vi "svx_DAQ_ConvertState_2000toCurrent.vi"(10 "State_2000":T8 {"Channel Info Array"."Channel Type" items=["Voltage (V)"=0, "Charge (C)"=9, "-"=99, "SPL (Pa)"=3, "Force (lbf)"=6, "Force (N)"=1, "Acceleration (g) - IEPE"=2, "Acceleration (g) - Charge"=12, "Acceleration (g) - 4 wire DC Voltage"=22, "Velocity (in/s)"=7, "Velocity (mm/s)"=8, "Prox Probe (mil)"=4, "Prox Probe (mm)"=5]}, 11 "Default Control State in":T9 caption="State" {"Timing Control 2" format="%#_6f"; "Channel Info Array"."Max" min=0.0 format="± %^#_4g"; "Channel Info Array"."Channel Type" items=["Voltage (V)"=0, "Charge (C)"=9, "-"=99, "SPL (Pa)"=3, "Force (lbf)"=6, "Force (N)"=1, "Acceleration (g) - IEPE"=2, "Acceleration (g) - Charge"=12, "Acceleration (g) - 4 wire DC Voltage"=22, "Velocity (in/s)"=7, "Velocity (mm/s)"=8, "Prox Probe (mil)"=4, "Prox Probe (mm)"=5]}) -> (3 "Default Control State out":T9 caption="State" {"Timing Control 2" format="%#_6f"; "Channel Info Array"."Max" min=0.0 format="± %^#_4g"; "Channel Info Array"."Channel Type" items=["Voltage (V)"=0, "Charge (C)"=9, "-"=99, "SPL (Pa)"=3, "Force (lbf)"=6, "Force (N)"=1, "Acceleration (g) - IEPE"=2, "Acceleration (g) - Charge"=12, "Acceleration (g) - 4 wire DC Voltage"=22, "Velocity (in/s)"=7, "Velocity (mm/s)"=8, "Prox Probe (mil)"=4, "Prox Probe (mm)"=5]})   [LabVIEW 2017, in "SVX NI-DAQmx AI Configuration XControl.xctl"]
uses:
  <vilib>/addons/Sound and Vibration/svt_DAQmx/Configuration XControl/SVX NI-DAQmx AI Configuration XControl.xctl
  <vilib>/addons/Sound and Vibration/svt_DAQmx/Configuration XControl/SubVIs/svx_DAQ_State.ctl
  <vilib>/addons/Sound and Vibration/svt_DAQmx/Configuration XControl/Controls/svx_DAQ_ChannelInfo.ctl
  <vilib>/addons/Sound and Vibration/svt_DAQmx/Configuration XControl/Controls/svx_DAQ_ChannelType.ctl
  <vilib>/addons/Sound and Vibration/svt_DAQmx/Configuration XControl/Controls/svx_DAQ_Coupling.ctl
  <vilib>/addons/Sound and Vibration/svt_DAQmx/Configuration XControl/Controls/svx_DAQ_Excitation.ctl
  <vilib>/addons/Sound and Vibration/svt_DAQmx/Configuration XControl/Controls/svx_DAQ_TimingType.ctl
  <vilib>/addons/Sound and Vibration/svt_DAQmx/Configuration XControl/Controls/svx_DAQ_ReferenceType.ctl
  <vilib>/addons/Sound and Vibration/svt_DAQmx/Configuration XControl/Controls/svx_DAQ_RotationDirection.ctl
  <vilib>/addons/Sound and Vibration/svt_DAQmx/Configuration XControl/Controls/svx_DAQ_Tach_Slope.ctl
  <vilib>/addons/Sound and Vibration/svt_DAQmx/Configuration XControl/Controls/svx_DAQ_Trigger_Slope.ctl
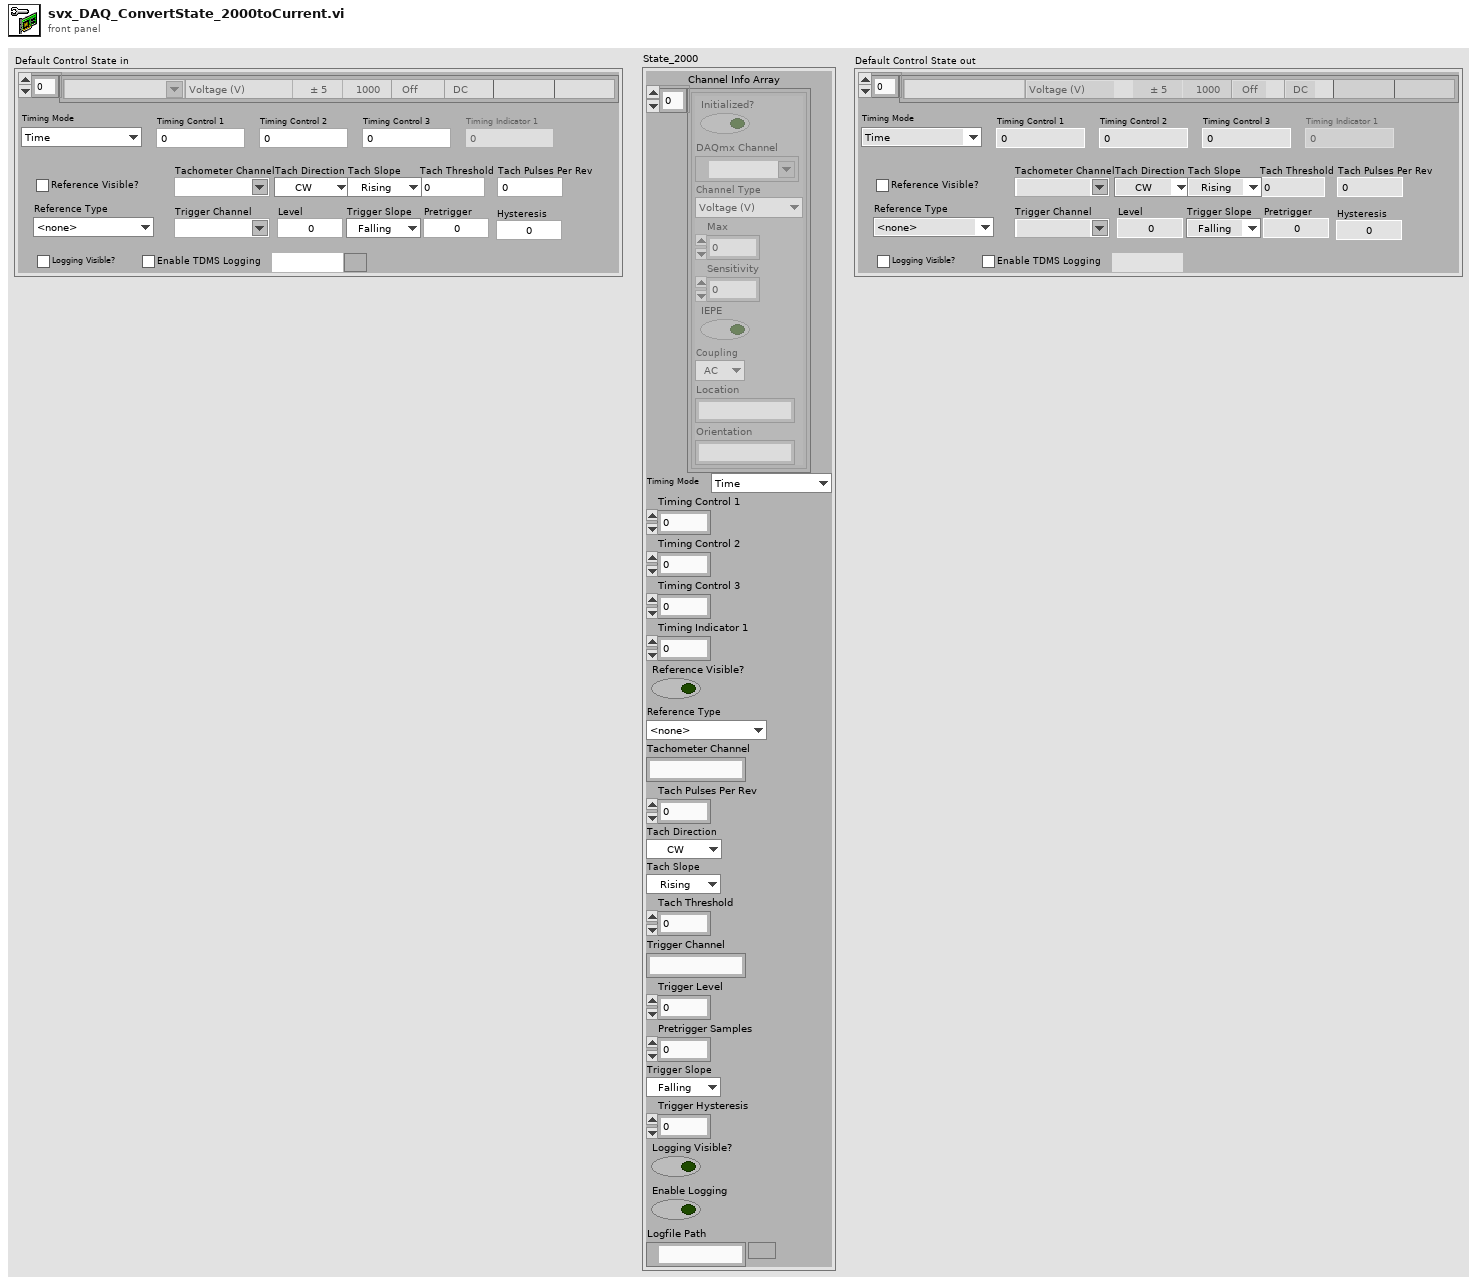
[diagram p1: front panel]
types:
  T1 = typedef "SVX NI-DAQmx AI Configuration XControl.xctl/svx_DAQ_ChannelType.ctl" = u16
  T2 = typedef "SVX NI-DAQmx AI Configuration XControl.xctl/svx_DAQ_Coupling.ctl" = enum16{"AC", "DC"}
  T3 = typedef "SVX NI-DAQmx AI Configuration XControl.xctl/svx_DAQ_TimingType.ctl" = enum16{"Time", "Frequency", "Order"}
  T4 = typedef "SVX NI-DAQmx AI Configuration XControl.xctl/svx_DAQ_ReferenceType.ctl" = enum16{"<none>", "Analog Tachometer", "Analog SW Trigger"}
  T5 = typedef "SVX NI-DAQmx AI Configuration XControl.xctl/svx_DAQ_RotationDirection.ctl" = enum16{"CW", "CCW"}
  T6 = typedef "SVX NI-DAQmx AI Configuration XControl.xctl/svx_DAQ_Tach_Slope.ctl" = enum16{"Rising", "Falling"}
  T7 = typedef "SVX NI-DAQmx AI Configuration XControl.xctl/svx_DAQ_Trigger_Slope.ctl" = enum16{"Falling", "Rising"}
  T8 = cluster{"Channel Info Array":cluster{"Initialized?":bool, "DAQmx Channel":tag, "Channel Type":T1, "Max":dbl, "Sensitivity":dbl, "IEPE":bool, "Coupling":T2, "Location":string, "Orientation":string}[], "Timing Mode":T3, "Timing Control 1":dbl, "Timing Control 2":dbl, "Timing Control 3":i32, "Timing Indicator 1":dbl, "Reference Visible?":bool, "Reference Type":T4, "Tachometer Channel":string, "Tach Pulses Per Rev":i32, "Tach Direction":T5, "Tach Slope":T6, "Tach Threshold":dbl, "Trigger Channel":string, "Trigger Level":dbl, "Pretrigger Samples":i32, "Trigger Slope":T7, "Trigger Hysteresis":dbl, "Logging Visible?":bool, "Enable Logging":bool, "Logfile Path":path}
  T9 = typedef "SVX NI-DAQmx AI Configuration XControl.xctl/svx_DAQ_State.ctl" = cluster{"Channel Info Array":T10[], "Timing Mode":T3, "Timing Control 1":dbl, "Timing Control 2":dbl, "Timing Control 3":i32, "Timing Indicator 1":dbl, "Reference Visible?":bool, "Reference Type":T4, "Tachometer Channel":string, "Tach Pulses Per Rev":i32, "Tach Direction":T5, "Tach Slope":T6, "Tach Threshold":dbl, "Trigger Channel":string, "Trigger Level":dbl, "Pretrigger Samples":i32, "Trigger Slope":T7, "Trigger Hysteresis":dbl, "Logging Visible?":bool, "Enable Logging":bool, "Logfile Path":path}
  T10 = typedef "SVX NI-DAQmx AI Configuration XControl.xctl/svx_DAQ_ChannelInfo.ctl" = cluster{"Initialized?":bool, "DAQmx Channel":tag, "Channel Type":T1, "Max":dbl, "Sensitivity":dbl, "Excitation":bool, "Coupling":T2, "Location":string, "Orientation":string, "excitation":T11}
  T11 = typedef "svx_DAQ_Excitation.ctl" = enum16{"Off", "Min", "Max"}
  T12 = cluster{"Initialized?":bool, "DAQmx Channel":tag, "Channel Type":T1, "Max":dbl, "Sensitivity":dbl, "IEPE":bool, "Coupling":T2, "Location":string, "Orientation":string}[]
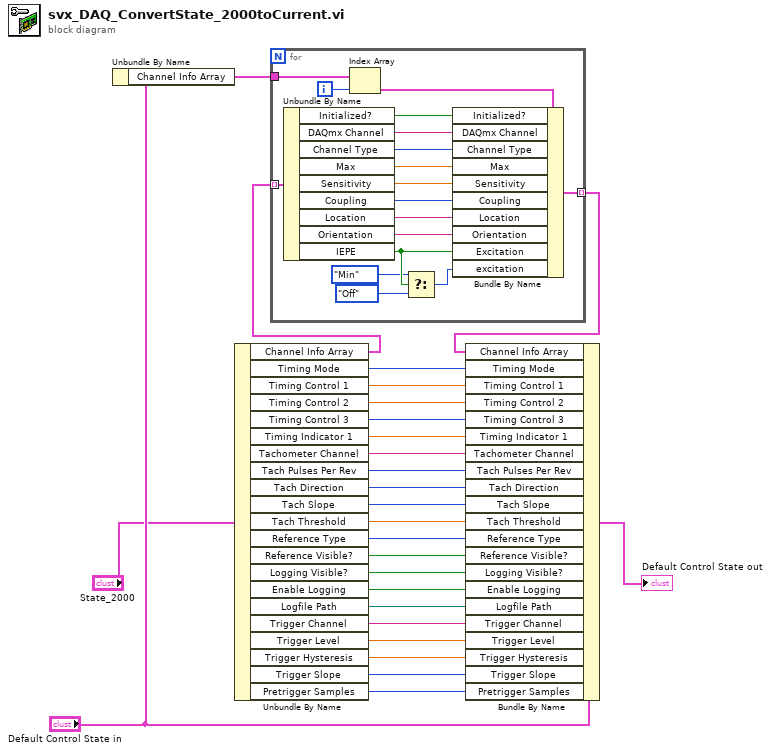
[diagram p0: block diagram]
diagram:
  n1 = Unbundle By Name("Default Control State in") -> ("Channel Info Array"=w15:T10[])
  n2 = Unbundle By Name("State_2000") -> ("Channel Info Array"=w13:T12, "Timing Mode"=w2:T3, "Timing Control 1"=w3:dbl, "Timing Control 2"=w4:dbl, "Timing Control 3"=w5:i32, "Timing Indicator 1"=w6:dbl, "Tachometer Channel"=w7:string, "Tach Pulses Per Rev"=w8:i32, "Tach Direction"=w9:T5, "Tach Slope"=w10:T6, "Tach Threshold"=w11:dbl, "Reference Type"=w17:T4, "Reference Visible?"=w18:bool, "Logging Visible?"=w19:bool, "Enable Logging"=w20:bool, "Logfile Path"=w21:path, "Trigger Channel"=w26:string, "Trigger Level"=w25:dbl, "Trigger Hysteresis"=w24:dbl, "Trigger Slope"=w23:T7, "Pretrigger Samples"=w22:i32)
  n3 = for {
    tunnel: w13 -> [w43] mode=indexing
    tunnel: w15 -> [w42]
    tunnel: [w27] -> w16 mode=indexing
    i -> [w41]
    n4 = Unbundle By Name(w43) -> ("Initialized?"=w39:bool, "DAQmx Channel"=w38:tag, "Channel Type"=w37:T1, "Max"=w36:dbl, "Sensitivity"=w35:dbl, "Coupling"=w34:T2, "Location"=w33:string, "Orientation"=w32:string, "IEPE"=w31:bool)
    n5 = Index Array(array=w42, index=w41) -> (element=w40:T10)
    n6 = Select(t=svx_DAQ_Excitation."Min" ("excitation"), s=w31, f=svx_DAQ_Excitation."Off" ("excitation")) -> (s? t:f=w28:T11)
    n7 = Bundle By Name(cluster=w40, "Initialized?"=w39, "DAQmx Channel"=w38, "Channel Type"=w37, "Max"=w36, "Sensitivity"=w35, "Coupling"=w34, "Location"=w33, "Orientation"=w32, "Excitation"=w31, "excitation"=w28) -> (w27:T10)
  }
  n8 = Bundle By Name(cluster="Default Control State in", "Channel Info Array"=w16, "Timing Mode"=w2, "Timing Control 1"=w3, "Timing Control 2"=w4, "Timing Control 3"=w5, "Timing Indicator 1"=w6, "Tachometer Channel"=w7, "Tach Pulses Per Rev"=w8, "Tach Direction"=w9, "Tach Slope"=w10, "Tach Threshold"=w11, "Reference Type"=w17, "Reference Visible?"=w18, "Logging Visible?"=w19, "Enable Logging"=w20, "Logfile Path"=w21, "Trigger Channel"=w26, "Trigger Level"=w25, "Trigger Hysteresis"=w24, "Trigger Slope"=w23, "Pretrigger Samples"=w22) -> (→"Default Control State out":T9)
